vi "Import DOS (DOSCAR) from DB.vi"(6 "Reference Energy/atom (pure Crystal) (eV)":dbl=-2.489625, 8 "error in (no error)":errorcluster, 9 "# of Atoms":i32, 10 "DOSCAR ID":string, 11 "connection reference":T3) -> (0 "error out":errorcluster, 1 "Extracted Parameters":T1, 2 "OSZICAR Raw":T2, 3 "connection reference out":T3)   [LabVIEW 2010]
uses:
  <vilib>/addons/database/Connection.llb/Conn ObjectReference.ctl
  <vilib>/addons/database/_DB Variant To Data/Database Variant To Data.xnode
  <vilib>/addons/database/NI_Database_API.lvlib
panel:
  out "Bulk Formation Energies Array (eV)":dbl[](array[numeric])
  out "Ionic Relaxation Energies Array (eV)":dbl[](array[numeric])
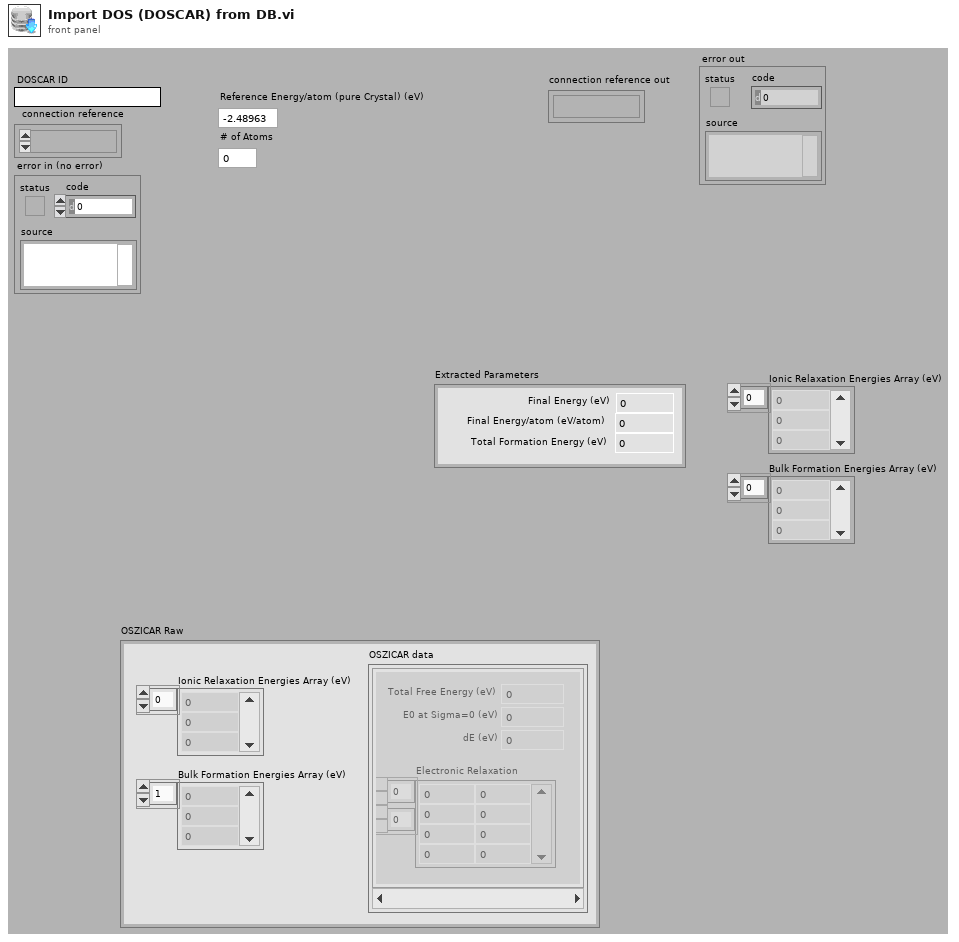
[diagram p1: front panel]
types:
  T1 = cluster{"Final Energy (eV)":dbl, "Final Energy/atom (eV/atom)":dbl, "Total Formation Energy (eV)":dbl}
  T2 = cluster{"OSZICAR data":cluster{"Total Free Energy (eV)":dbl, "E0 at Sigma=0 (eV)":dbl, "dE (eV)":dbl, "Electronic Relaxation":dbl[][]}[], "Ionic Relaxation Energies Array (eV)":dbl[], "Bulk Formation Energies Array (eV)":dbl[]}
  T3 = typedef "NI_Database_API.lvlib/Conn ObjectReference.ctl" = refnum<k1>
  T4 = cluster{"Total Free Energy (eV)":dbl, "E0 at Sigma=0 (eV)":dbl, "dE (eV)":dbl, "Electronic Relaxation":dbl[][]}[]
  T5 = cluster{"OSZICAR data":cluster{"Total Free Energy (eV)":dbl, "E0 at Sigma=0 (eV)":dbl, "dE (eV)":dbl, "Electronic Relaxation":dbl[][]}[], dbl[], dbl[]}
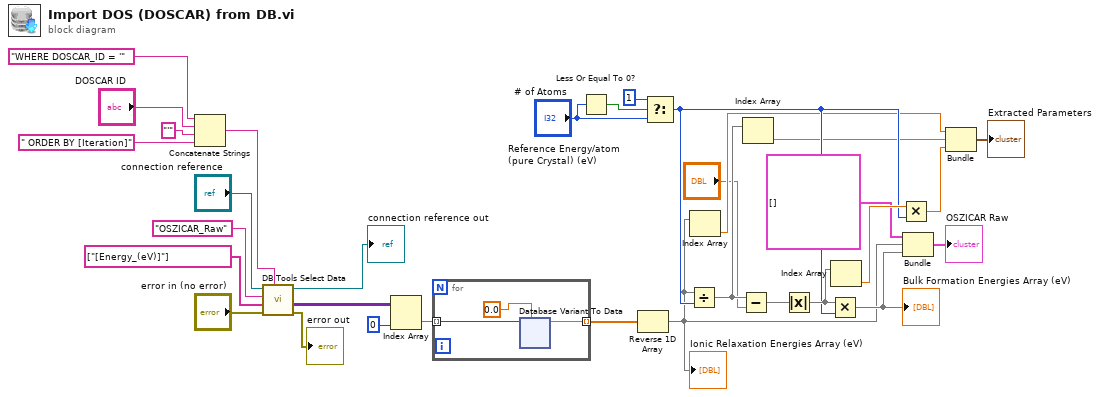
[diagram p0: block diagram]
diagram:
  n1 = Concatenate Strings("WHERE DOSCAR_ID = '", "DOSCAR ID", "'" ("string"), " ORDER BY [Iteration]" ("string")) -> (w25:string)
  n2 = call <vilib>:"DB Tools Select Data.vi"("condition"=w25, "error in (no error)"="error in (no error)", "columns"=string[] ["[Energy_(eV)]"], "table"="OSZICAR_Raw", "connection reference"="connection reference") -> ("error out"=→"error out":errorcluster, "data"=w26:variant[][], "connection reference out"=→"connection reference out":T3)  [unwired: 1 in]
  n3 = Index Array(array=w26, index (col)=0 ("index (row)")) -> (element=w11:variant[])  [unwired: 1 in]
  n4 = for {
    tunnel: w11 -> [w35] mode=indexing
    tunnel: [w34] -> w2 mode=indexing
    n5 = xnode "Database Variant To Data"("database variant"=w35, "type"=0.0) -> ("data"=w34:dbl)  [unwired: 1 in, 1 out]
  }
  n6 = Less Or Equal To 0?(x="# of Atoms") -> (x <= 0?=w21:bool)
  n7 = Reverse 1D Array(array=w2) -> (reversed array=w1:dbl[])
  "Ionic Relaxation Energies Array (eV)" <- w1
  n8 = Select(t=1, s=w21, f="# of Atoms") -> (s? t:f=w18:i32)
  n9 = Divide(x=w1, y=w18) -> (x/y=w17:dbl[])
  n10 = Index Array(array=w1) -> (element=w16:dbl)  [unwired: 1 in]
  n11 = Subtract(x=w17, y="Reference Energy/atom (pure Crystal) (eV)") -> (x-y=w23:dbl[])
  n12 = Index Array(array=w17) -> (element=w15:dbl)  [unwired: 1 in]
  n13 = Absolute Value(x=w23) -> (abs(x)=w19:dbl[])
  n14 = Multiply(x=w19, y=w18) -> (x*y=w5:dbl[])
  "Bulk Formation Energies Array (eV)" <- w5
  n15 = Index Array(array=w19) -> (element=w22:dbl)  [unwired: 1 in]
  n16 = Multiply(x=w22, y=w18) -> (x*y=w14:dbl)
  n17 = Bundle("OSZICAR data"=T4 [], w1, w5) -> (→"OSZICAR Raw":T5)  [unwired: 1 in]
  n18 = Bundle("data"=w16, w15, w14) -> (→"Extracted Parameters":cluster{"data":dbl, dbl, dbl})  [unwired: 1 in]
